vi "TSPopup.String to Variant Value.vi"(8 "error in (no error)":errorcluster, 10 "Cell String":string, 11 "Popup Parameters":T1) -> (0 "error out":errorcluster, 2 "Variant Value":variant, 3 "Popup Parameters out":T1)   [LabVIEW 2013]
doc: "Converts a string (as from a control's cell) to the proper value, using the popup parameters. Output as a variant.\n\nType Sensitive Popup \nCopyright © 2007, J. David Saunders\nAll rights reserved."
uses:
  TSPopup.Popup Call Parameters.ctl
  TSPopup.Data Type.ctl
panel:
  # "Type Sensitive Popup \nCopyright © 2007, J. David Saunders\nAll rights reserved."
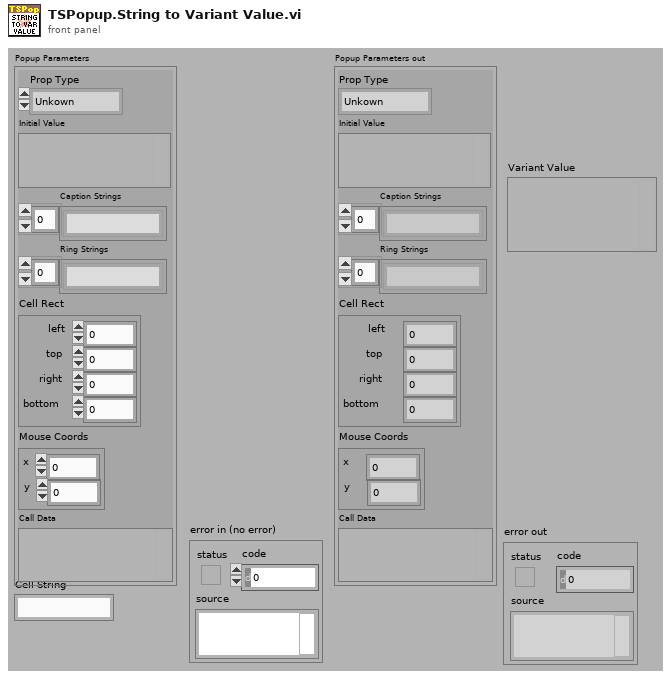
[diagram p1: front panel]
types:
  T1 = typedef "TSPopup.Popup Call Parameters.ctl" = cluster{"Prop Type":T2, "Initial Value":variant, "Caption Strings":string[], "Ring Strings":string[], "Cell Rect":cluster{"left":i16, "top":i16, "right":i16, "bottom":i16}, "Mouse Coords":cluster{"x":i16, "y":i16}, "Call Data":variant}
  T2 = typedef "TSPopup.Data Type.ctl" = enum16{"Unkown", "NO POPUP", "String", "Integer", "Float", "Color", "Boolean", "Ring", "Captioned String", "Captioned Integer", "Button Color", "2 Int Cluster", "4 Int Cluster"}
  T3 = cluster{"default value 1":i32, "default value 1":i32}
  T4 = cluster{"default value 1":i32, "default value 1":i32, "default value 1":i32, "default value 1":i32}
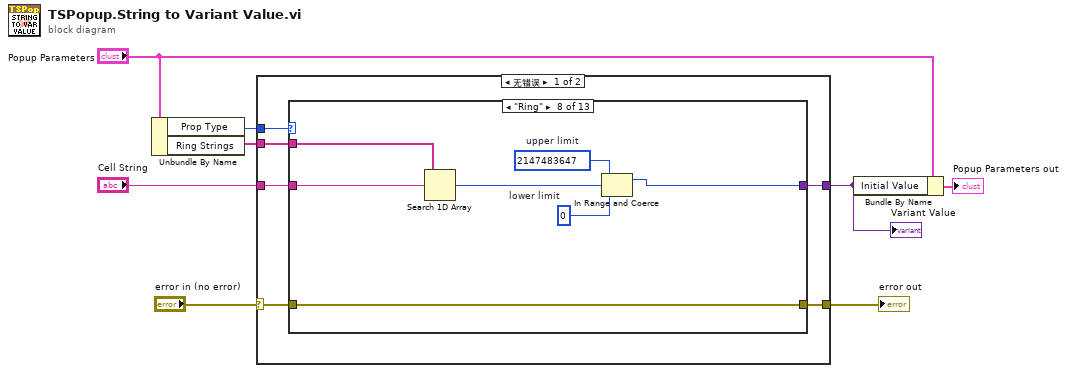
[diagram p0: block diagram]
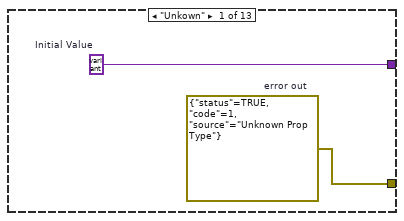
[diagram p2: hidden frame]
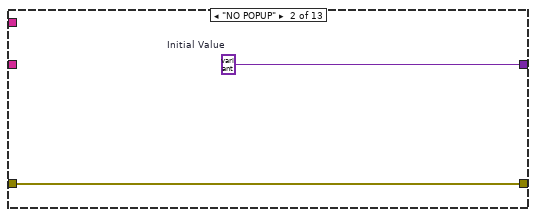
[diagram p3: hidden frame]
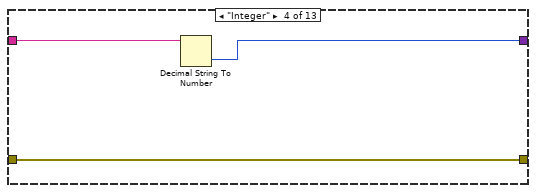
[diagram p5: hidden frame]
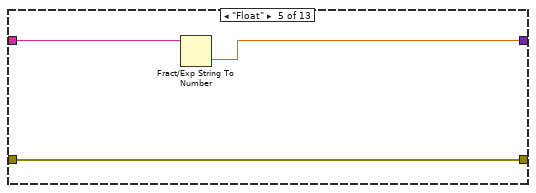
[diagram p6: hidden frame]
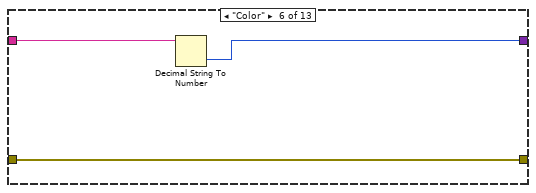
[diagram p7: hidden frame]
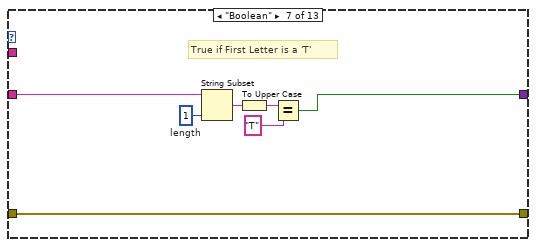
[diagram p8: hidden frame]
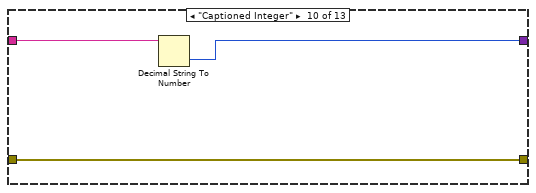
[diagram p10: hidden frame]
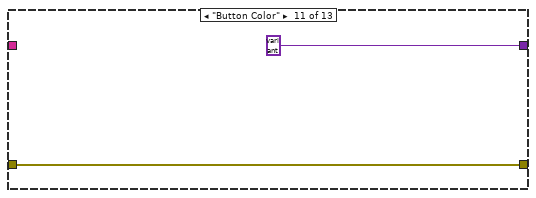
[diagram p11: hidden frame]
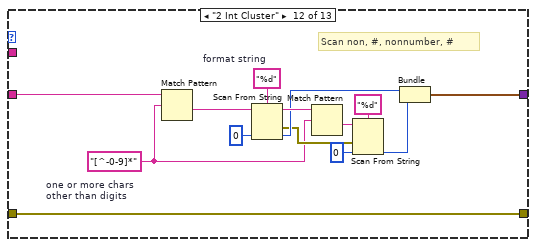
[diagram p12: hidden frame]
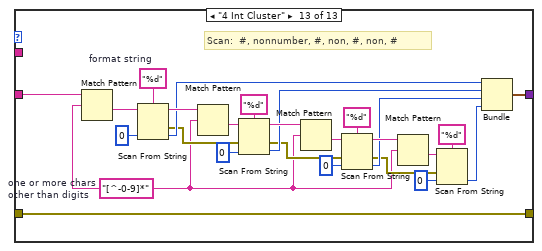
[diagram p13: hidden frame]
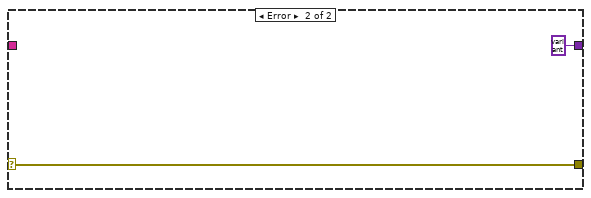
[diagram p14: hidden frame]
diagram:
  n1 = Unbundle By Name("Popup Parameters") -> ("Prop Type"=w8:T2, "Ring Strings"=w5:string[])
  n2 = case shown="无错误" "error in (no error)" {
    selector: "error in (no error)" -> [w11 w92]
    tunnel: w8 -> [w12 _]
    tunnel: "Cell String" -> [w14 _]
    tunnel: w5 -> [w13 _]
    tunnel: [w9 w92] -> w4
    tunnel: [w10 variant] -> w2
    frame No Error {
      n3 = case shown="\"Ring\"" w12 {
        tunnel: [w16 w18 w20 w22 w25 w28 w31 w37 w45 w47 variant w57 w84] -> w10
        tunnel: w14 -> [_ _ w20 w23 w26 w29 w36 w42 w45 w48 _ w52 w67]
        tunnel: w13 -> [_ _ _ _ _ _ _ w43 _ _ _ _ _]
        tunnel: w11 -> [_ w17 w19 w21 w24 w27 w30 w41 w44 w46 w49 w54 w68]
        tunnel: [w15 w17 w19 w21 w24 w27 w30 w41 w44 w46 w49 w54 w68] -> w9
        frame "Unkown" {
          w15 = errorcluster {"status"=TRUE, "code"=1, "source"="Unknown Prop Type"}  # error out
          w16 = variant  # Initial Value
        }
        frame "NO POPUP" {
          w18 = variant  # Initial Value
        }
        frame "String" {
        }
        frame "Integer" {
          n4 = Decimal String To Number(string=w23) -> (number=w22:i32)  [unwired: 2 in, 1 out]
        }
        frame "Float" {
          n5 = Fract/Exp String To Number(string=w26) -> (number=w25:dbl)  [unwired: 3 in, 1 out]
        }
        frame "Color" {
          n6 = Decimal String To Number(string=w29) -> (number=w28:i32)  [unwired: 2 in, 1 out]
        }
        frame "Boolean" {
          w35 = 1  # length
          # "True if First Letter is a 'T'"
          n7 = String Subset(string=w36, length (rest)=w35) -> (substring=w34:string)  [unwired: 1 in]
          n8 = To Upper Case(1:w34) -> (0:w33:string)
          n9 = Equal?(x=w33, y="T") -> (x = y?=w31:bool)
        }
        frame "Ring" {
          w39 = 0  # lower limit
          w40 = 2147483647  # upper limit
          n10 = Search 1D Array(1D array=w43, element=w42) -> (index of element=w38:i32)  [unwired: 1 in]
          n11 = In Range and Coerce(upper limit=w40, x=w38, lower limit=w39) -> (coerced(x)=w37:i32)  [unwired: 1 out]
        }
        frame "Captioned String" {
        }
        frame "Captioned Integer" {
          n12 = Decimal String To Number(string=w48) -> (number=w47:i32)  [unwired: 2 in, 1 out]
        }
        frame "Button Color" {
        }
        frame "2 Int Cluster" {
          w51 = "[^-0-9]*"  # one or more chars other than digits
          w64 = "%d"  # format string
          # "Scan non, #, nonnumber, #"
          n13 = Match Pattern(string=w52, regular expression=w51) -> (after substring=w53:string)  [unwired: 1 in, 3 out]
          n14 = Scan From String(format string=w64, input string=w53, default 1=0 ("default value 1")) -> (remaining string=w62:string, error out=w55:errorcluster, output 1=w56:i32)  [unwired: 2 in, 1 out]
          n15 = Match Pattern(string=w62, regular expression=w51) -> (after substring=w59:string)  [unwired: 1 in, 3 out]
          n16 = Scan From String(format string="%d", input string=w59, error in=w55, default 1=0 ("default value 1")) -> (output 1=w58:i32)  [unwired: 1 in, 3 out]
          n17 = Bundle("default value 1"=w56, "default value 1"=w58) -> (w57:T3)  [unwired: 1 in]
        }
        frame "4 Int Cluster" {
          w65 = "[^-0-9]*"  # one or more chars other than digits
          w90 = "%d"  # format string
          # "Scan:  #, nonnumber, #, non, #, non, #"
          n18 = Match Pattern(string=w67, regular expression=w65) -> (after substring=w66:string)  [unwired: 1 in, 3 out]
          n19 = Scan From String(format string=w90, input string=w66, default 1=0 ("default value 1")) -> (remaining string=w88:string, error out=w71:errorcluster, output 1=w83:i32)  [unwired: 2 in, 1 out]
          n20 = Match Pattern(string=w88, regular expression=w65) -> (after substring=w85:string)  [unwired: 1 in, 3 out]
          n21 = Scan From String(format string="%d", input string=w85, error in=w71, default 1=0 ("default value 1")) -> (remaining string=w76:string, error out=w70:errorcluster, output 1=w73:i32)  [unwired: 1 in, 1 out]
          n22 = Match Pattern(string=w76, regular expression=w65) -> (after substring=w82:string)  [unwired: 1 in, 3 out]
          n23 = Scan From String(format string="%d", input string=w82, error in=w70, default 1=0 ("default value 1")) -> (remaining string=w75:string, error out=w69:errorcluster, output 1=w72:i32)  [unwired: 1 in, 1 out]
          n24 = Match Pattern(string=w75, regular expression=w65) -> (after substring=w77:string)  [unwired: 1 in, 3 out]
          n25 = Scan From String(format string="%d", input string=w77, error in=w69, default 1=0 ("default value 1")) -> (output 1=w74:i32)  [unwired: 1 in, 3 out]
          n26 = Bundle("default value 1"=w83, "default value 1"=w73, "default value 1"=w72, "default value 1"=w74) -> (w84:T4)  [unwired: 1 in]
        }
      }
    }
    frame Error {
    }
  }
  "error out" <- w4
  "Variant Value" <- w2
  n27 = Bundle By Name(cluster="Popup Parameters", "Initial Value"=w2) -> (→"Popup Parameters out":T1)
